vi "EMBALLAGE_BDD_FichiersSQLEnregistres.vi"(8 "Error in":errorcluster caption="Error in (no error)") -> (0 "Error out":errorcluster, 3 "Dans la gamme ?":bool)   [LabVIEW 2020]
uses:
  <vilib>/Utility/miscctls.llb/LVDateTimeRec.ctl
  Modules/FS/60_FS_Controles/60_FS_SetGet.ctl
panel:
  out "horodatage":timestamp
  out "cluster date/heure":T1
  out "temps actuel":timestamp
  out "dernière modif.":timestamp
  out "noms des fichiers":string[](array[string])
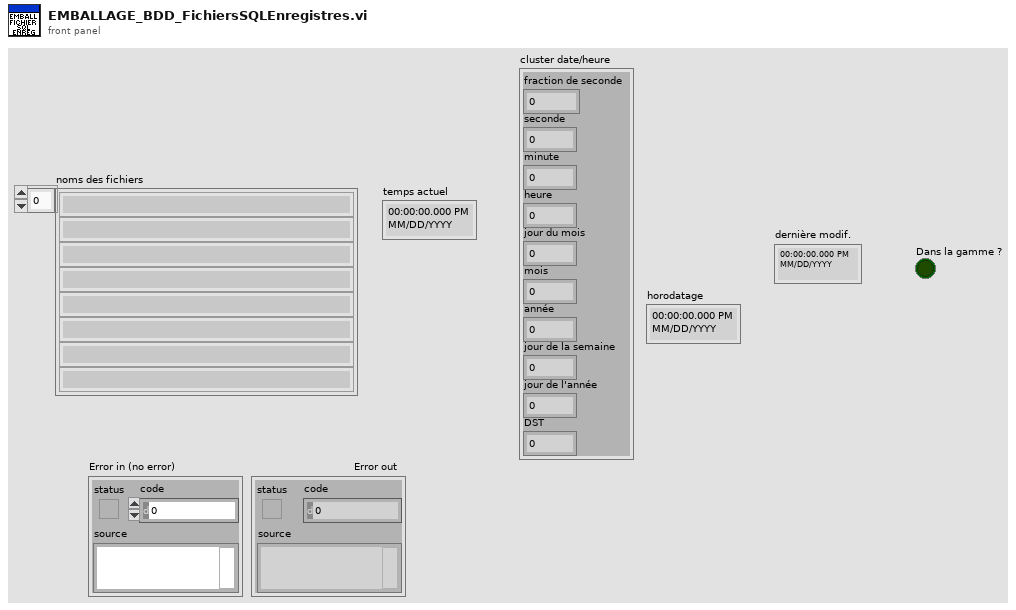
[diagram p1: front panel]
types:
  T1 = typedef "LVDateTimeRec.ctl" = cluster{"fractional second":dbl, "second":i32, "minute":i32, "hour":i32, "day of month":i32, "month":i32, "year":i32, "day of week":i32, "day of year":i32, "DST":i32}
  T2 = typedef "60_FS_SetGet.ctl" = enum16{"set", "get"}
  T3 = typedef "60_FS_CLT_Chemins.ctl" = cluster{"Racine_local":path, "Racine_reseau":path, "Racine_Support_Application":path, "Fichier_Journalisation":path, "Connexion_BDD_VSX":path, "Connexion_BDD_PLZ":path}
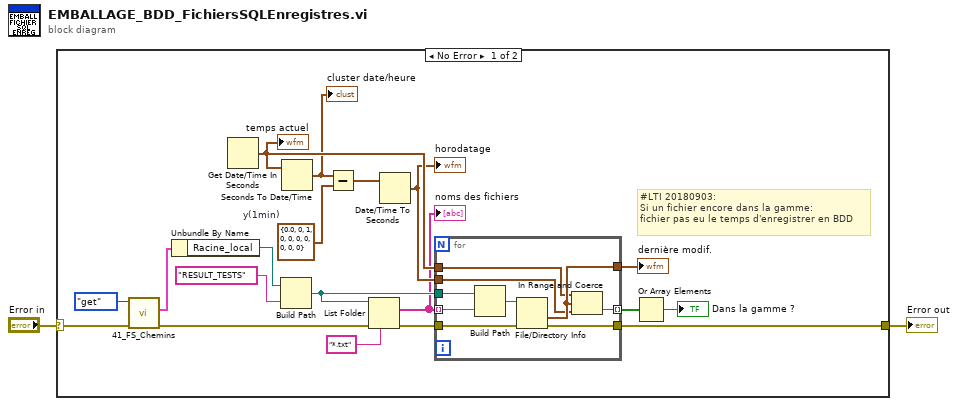
[diagram p0: block diagram]
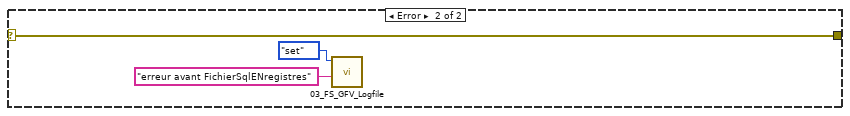
[diagram p2: hidden frame]
diagram:
  n1 = case shown="No Error" "Error in" {
    selector: "Error in" -> [w4 w33]
    tunnel: [w3 w33] -> w1
    frame No Error {
      w10 = T1 {"fractional second"=0.0, "second"=0, "minute"=1, "hour"=0, "day of month"=0, "month"=0, "year"=0, "day of week"=0, "day of year"=0, "DST"=0}  # y(1min)
      # "#LTI 20180903:\nSi un fichier encore dans la gamme:\nfichier pas eu le temps d'enregistrer en BDD"
      n2 = call "41_FS_Chemins.vi"("error in (no error)"=w4, "SetGet"=60_FS_SetGet."get") -> ("error out"=w16:errorcluster, "CLT_Chemins_out"=w20:T3)  [unwired: 8 in]
      n3 = Unbundle By Name(w20) -> ("Racine_local"=w19:path)
      n4 = Get Date/Time In Seconds() -> (seconds since 1Jan1904=w12:timestamp)
      "temps actuel" <- w12
      n5 = Build Path(base path=w19, name or relative path="RESULT_TESTS" ("chemin de base")) -> (appended path=w15:path)
      n6 = Seconds To Date/Time(time stamp (now)=w12) -> (date time rec=w11:T1)  [unwired: 1 in]
      "cluster date/heure" <- w11
      n7 = Subtract(x=w11, y=w10) -> (x-y=w9:T1)
      n8 = List Folder(path=w15, pattern="*.txt" ("filtre"), error in=w16) -> (filenames=w6:string[], error out=w14:errorcluster)  [unwired: 1 in, 2 out]
      "noms des fichiers" <- w6
      n9 = Date/Time To Seconds(2:w9) -> (0:w8:timestamp)  [unwired: 1 in]
      "horodatage" <- w8
      n10 = for {
        tunnel: w15 -> [w30]
        tunnel: w14 -> [w28]
        tunnel: [w27] -> w13
        tunnel: w12 -> [w26]
        tunnel: w8 -> [w25]
        tunnel: [w24] -> w7 mode=indexing
        tunnel: w6 -> [w23] mode=indexing
        tunnel: [w22] -> w3
        n11 = Build Path(base path=w30, name or relative path=w23) -> (appended path=w29:path)
        n12 = File/Directory Info(path=w29, error in=w28) -> (last mod=w27:timestamp, error out=w22:errorcluster)  [unwired: 5 out]
        n13 = In Range and Coerce(upper limit=w26, x=w27, lower limit=w25) -> (In Range?=w24:bool)  [unwired: 1 out]
      }
      "dernière modif." <- w13
      n14 = Or Array Elements(Boolean array=w7) -> (logical OR=→"Dans la gamme ?":bool)
    }
    frame Error {
      n15 = call "03_FS_GFV_Logfile.vi"("Chaîne"="erreur avant FichierSqlENregistres", "States"=60_FS_SetGet."set") -> ()  [unwired: 8 in, 2 out]
    }
  }
  "Error out" <- w1
